vi "final Vi.vi"() -> ()   [LabVIEW 2018]
uses:
  <vilib>/Utility/file.llb/Read Delimited Spreadsheet (string).vi
  <vilib>/Utility/file.llb/Read Delimited Spreadsheet (DBL).vi
  <vilib>/Analysis/3filter.llb/Equi-Ripple BandPass (DBL).vi
  <vilib>/Analysis/NI_AALBase.lvlib
  <vilib>/Analysis/NI_AAL_SigProc.lvlib
panel:
  out "Locations 2":dbl[](array[numeric])
  out "yeee":dbl[](array[numeric])
  out "我們計算的RR":cluster{i32[], dbl[]}(graph)
  out "Array":dbl[](array[numeric])
  in  "threshold":dbl=10000.0 format="%0.2f"
  out "Locations":dbl[](array[numeric])
  in  "filter higher  stop freq":dbl(slide)=0.4094594594594595 scale=0.4..0.5
  out "平均心跳/分鐘":dbl
  out "?":bool
  out "RMSSD(ms)":dbl
  out "HR":cluster{i32[], dbl[]}[](graph)
  out "Mean R-R interval":dbl
  out "RR":cluster{dbl[], dbl[]}(graph)
  in  "filter lower stop freq":dbl(slide)=0.032972972972972976 scale=0.0..0.1
  out "Band filter":cluster{dbl[], "Filtered X":dbl[]}[](graph)
  out "Origin ECG":cluster{dbl[], i32[]}(graph)
  # "RMSSD越大，\n表示副交感神經作用越強"
  # "一般正常心跳約為50~100下/分鐘"
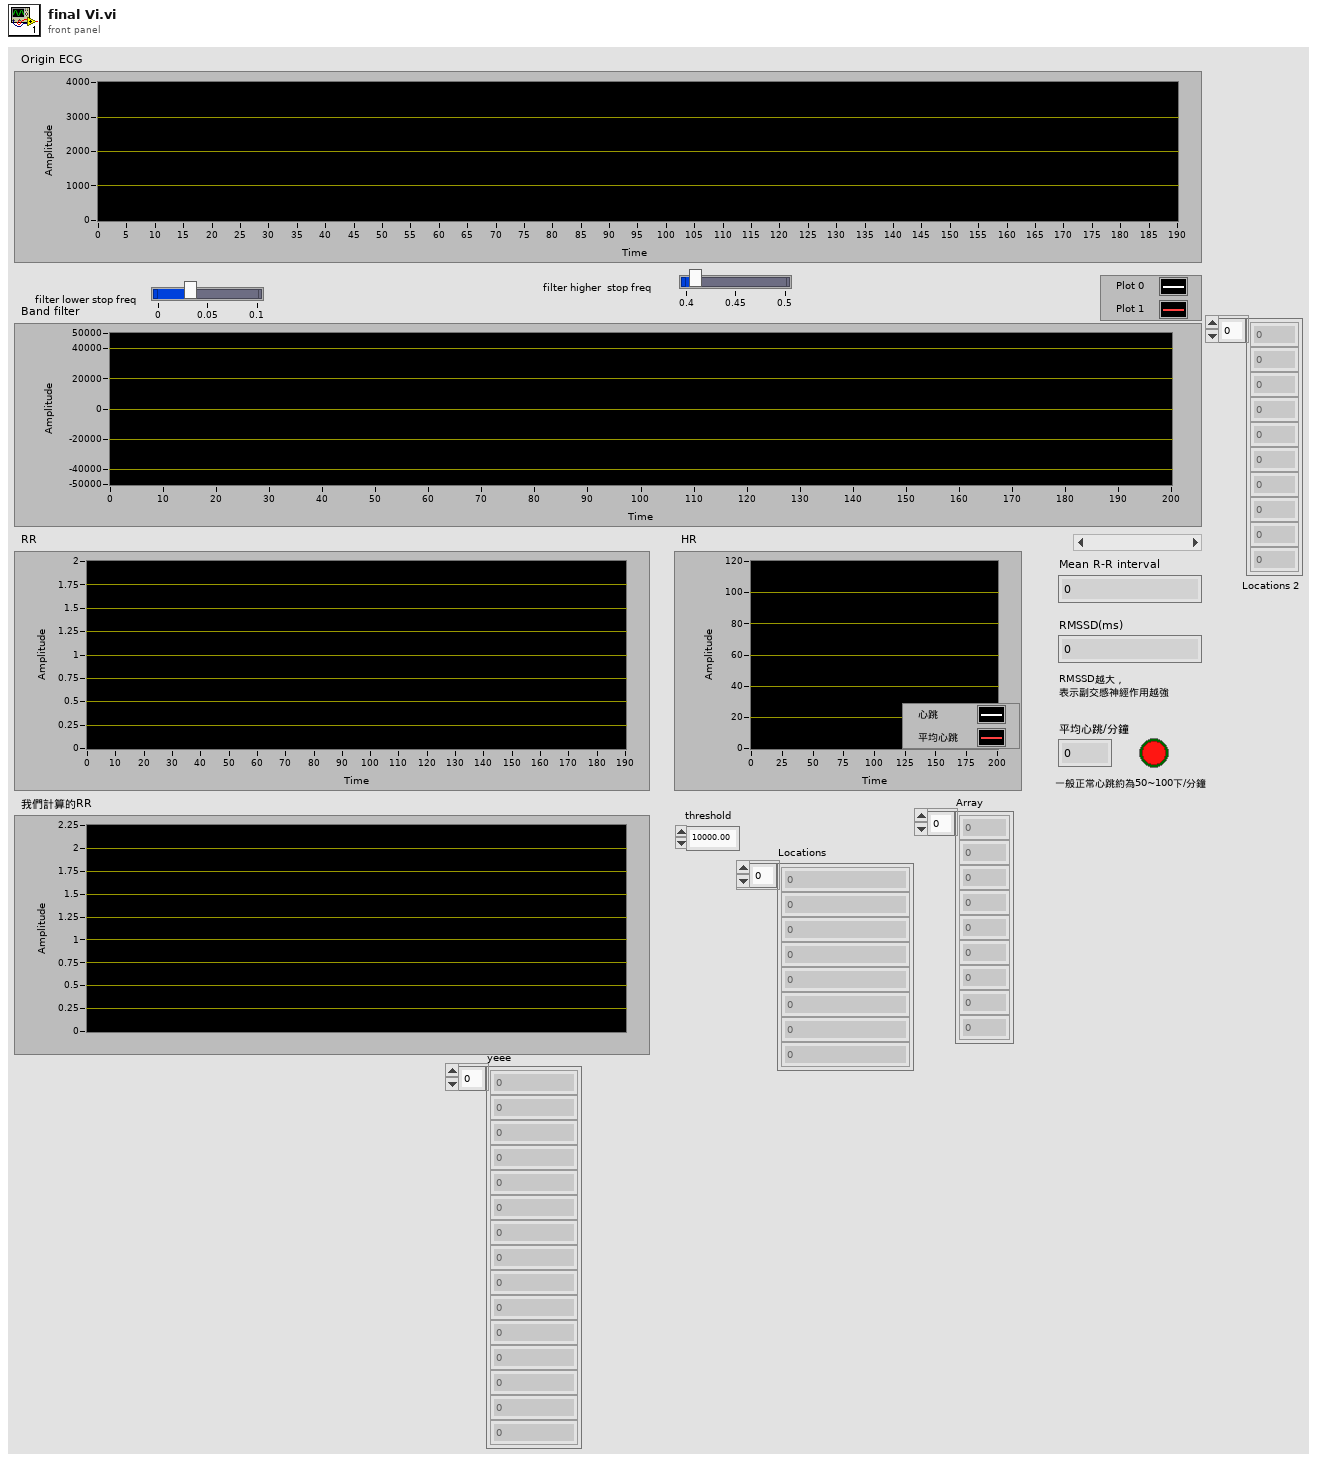
[diagram p1: front panel]
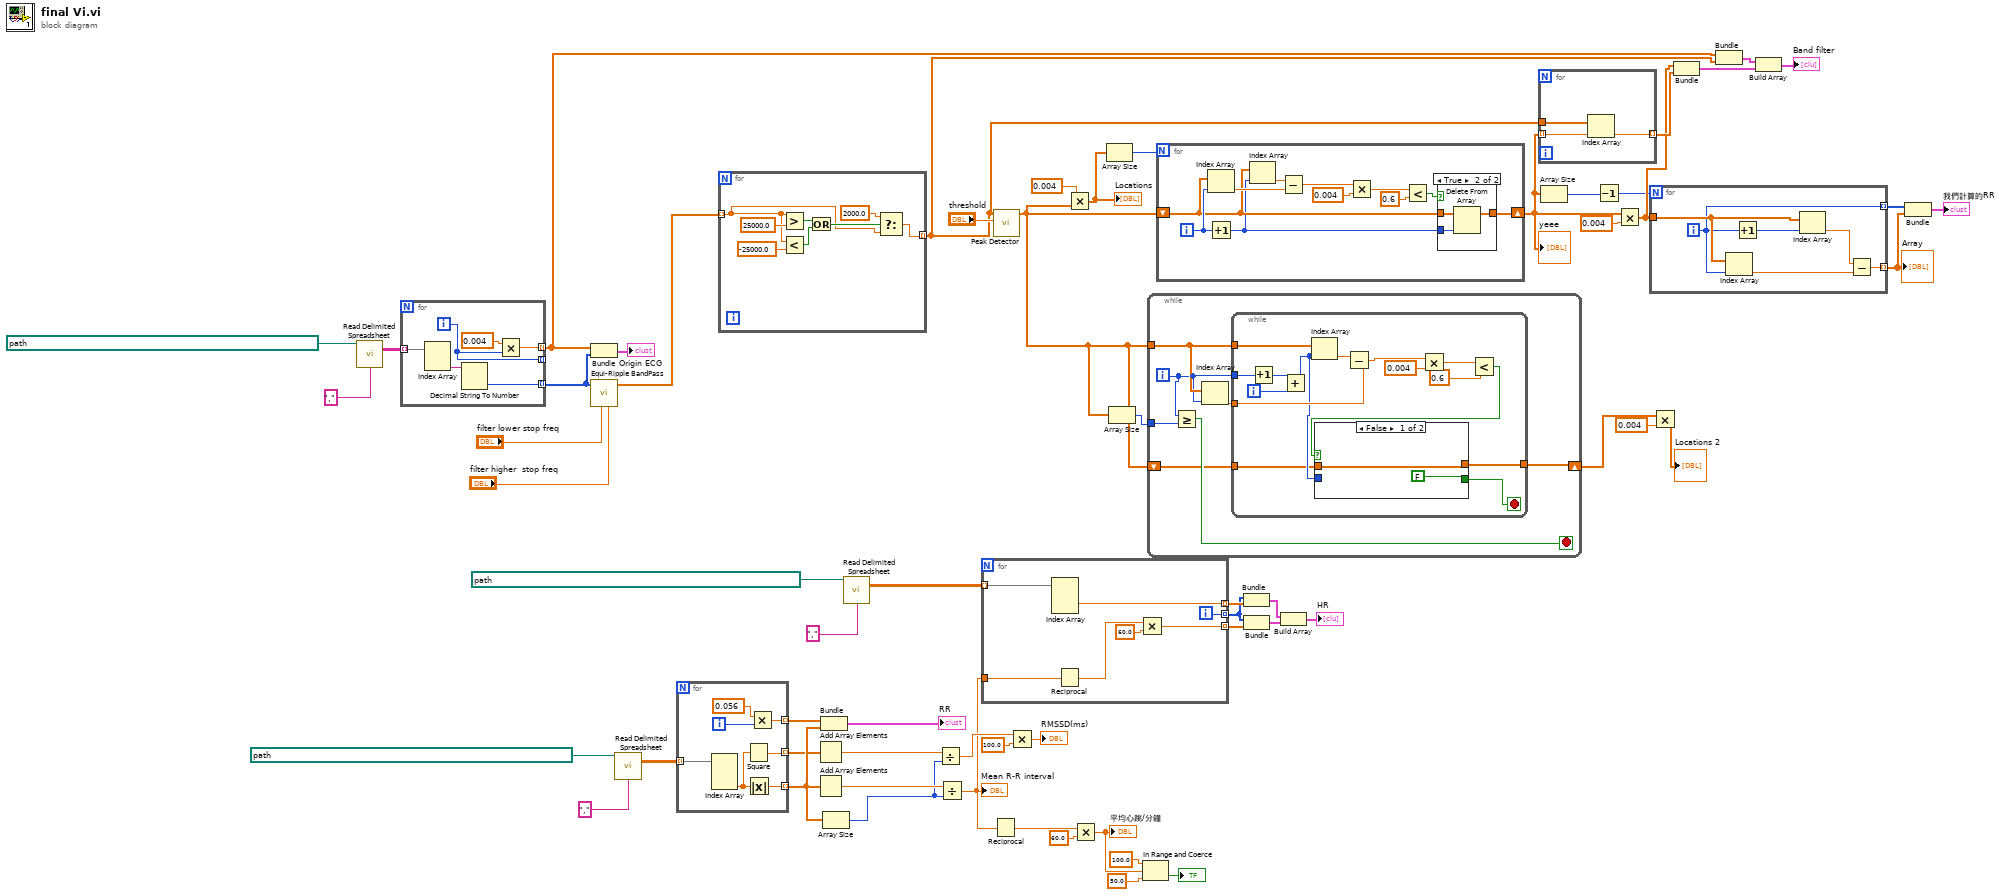
[diagram p0: block diagram]
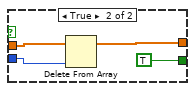
[diagram p2: hidden frame]
diagram:
  n1 = call-poly <vilib>:"Read Delimited Spreadsheet.vi"("file path (dialog if empty)"=path "D:/Documents/生醫儀表/data/2019_05_25__16_08_04_ECG.csv", "delimiter (\\t)"="," ("delimiter (\\t)")) -> ("all rows"=w59:string[][])  [unwired: 8 in, 5 out]
  n2 = for {
    tunnel: w59 -> [w66] mode=indexing
    tunnel: [w65] -> w23 mode=indexing
    tunnel: [w63] -> w17 mode=indexing
    tunnel: [w61] -> _ mode=indexing
    i -> [w61]
    n3 = Index Array(array=w66) -> (element #2=w62:string)  [unwired: 2 in, 1 out]
    n4 = Decimal String To Number(string=w62) -> (number=w65:i32)  [unwired: 2 in, 1 out]
    n5 = Multiply(x=0.004 ("y"), y=w61) -> (x*y=w63:dbl)
  }
  n6 = Bundle(w17, w23) -> (→"Origin ECG":cluster{dbl[], i32[]})  [unwired: 1 in]
  n7 = call-poly <vilib>:"Equi-Ripple BandPass.vi"("X"=w23, "lower stop freq"="filter lower stop freq", "higher stop freq"="filter higher  stop freq") -> ("Filtered X"=w9:dbl[])  [unwired: 5 in, 1 out]
  n8 = call-poly <vilib>:"Read Delimited Spreadsheet.vi"("file path (dialog if empty)"=path "D:/Documents/生醫儀表/data/2019_05_25__16_08_04_BR_RR.csv", "delimiter (\\t)"="," ("delimiter (\\t)")) -> ("all rows"=w56:dbl[][])  [unwired: 8 in, 5 out]
  n9 = for {
    tunnel: w56 -> [w73] mode=indexing
    tunnel: [w70] -> w54 mode=indexing
    tunnel: [w69] -> w50 mode=indexing
    tunnel: [w67] -> w40 mode=indexing
    i -> [w72]
    n10 = Index Array(array=w73) -> (element #3=w68:dbl)  [unwired: 3 in, 2 out]
    n11 = Square(x=w68) -> (x^2=w67:dbl)
    n12 = Absolute Value(x=w68) -> (abs(x)=w69:dbl)
    n13 = Multiply(x=0.056 ("y"), y=w72) -> (x*y=w70:dbl)
  }
  n14 = for {
    tunnel: w9 -> [w75] mode=indexing
    tunnel: [w74] -> w8 mode=indexing
    n15 = Greater?(x=w75, y=25000.0) -> (0:w79:bool)
    n16 = Less?(x=w75, y=-25000.0) -> (x < y?=w78:bool)
    n17 = Or(x=w79, y=w78) -> (x .or. y?=w77:bool)
    n18 = Select(t=2000.0, s=w77, f=w75) -> (s? t:f=w74:dbl)
  }
  n19 = Add Array Elements(numeric array=w40) -> (sum=w39:dbl)
  n20 = Add Array Elements(numeric array=w50) -> (sum=w51:dbl)
  n21 = Bundle(w54, w50) -> (→"RR":cluster{dbl[], dbl[]})  [unwired: 1 in]
  n22 = Array Size(array=w50) -> (size(s)=w38:i32)
  n23 = call-poly <vilib>:"Read Delimited Spreadsheet.vi"("file path (dialog if empty)"=path "D:/Documents/生醫儀表/data/2019_05_25__16_08_04_General.csv", "delimiter (\\t)"="," ("delimiter (\\t)")) -> ("all rows"=w47:dbl[][])  [unwired: 8 in, 5 out]
  n24 = Divide(x=w39, y=w38) -> (x/y=w37:dbl)
  n25 = Divide(x=w51, y=w38) -> (x/y=w32:dbl)
  "Mean R-R interval" <- w32
  n26 = for {
    tunnel: w47 -> [w88] mode=indexing
    tunnel: [w87] -> w46 mode=indexing
    tunnel: [w86] -> w45 mode=indexing
    tunnel: w32 -> [w85]
    tunnel: [w82] -> w41 mode=indexing
    i -> [w86]
    n27 = Index Array(array=w88) -> (element #2=w87:dbl)  [unwired: 3 in, 2 out]
    n28 = Reciprocal(x=w85) -> (1/x=w84:dbl)
    n29 = Multiply(x=w84, y=60.0) -> (x*y=w82:dbl)
  }
  n30 = Reciprocal(x=w32) -> (1/x=w34:dbl)
  n31 = call <vilib>:"Peak Detector.vi"("threshold"="threshold", "X"=w8) -> ("Locations"=w4:dbl[])  [unwired: 5 in, 4 out]
  n32 = Multiply(x=w37, y=100.0) -> (x*y=→"RMSSD(ms)":dbl)
  n33 = Multiply(x=0.004 ("y"), y=w4) -> (x*y=w14:dbl[])
  "Locations" <- w14
  n34 = Multiply(x=w34, y=60.0) -> (x*y=w31:dbl)
  "平均心跳/分鐘" <- w31
  n35 = Array Size(array=w14) -> (size(s)=w15:i32)
  n36 = Array Size(array=w4) -> (size(s)=w5:i32)
  n37 = In Range and Coerce(upper limit=100.0, x=w31, lower limit=50.0) -> (In Range?=→"?":bool)  [unwired: 1 out]
  n38 = while {
    tunnel: w4 -> [w94]
    tunnel: w5 -> [w92]
    shift-right: [w89] -> w2
    shift-left: w4 -> [w90]
    i -> [w93]
    stop <- w91 stop-if-true
    n39 = Greater Or Equal?(x=w93, y=w92) -> (x >= y?=w91:bool)
    n40 = Index Array(array=w94, index=w93) -> (element=w95:dbl)
    n41 = while {
      tunnel: w95 -> [w106]
      tunnel: w93 -> [w109]
      tunnel: w94 -> [w107]
      tunnel: w90 -> [w98]
      tunnel: [w97] -> w89
      i -> [w110]
      stop <- w96 stop-if-true
      n42 = Increment(x=w109) -> (x+1=w108:i32)
      n43 = Add(x=w108, y=w110) -> (x+y=w99:i32)
      n44 = Index Array(array=w107, index=w99) -> (element=w105:dbl)
      n45 = Subtract(x=w105, y=w106) -> (x-y=w101:dbl)
      n46 = Multiply(x=w101, y=0.004) -> (x*y=w104:dbl)
      n47 = Less?(x=w104, y=0.6) -> (x < y?=w100:bool)
      n48 = case shown="False" w100 {
        tunnel: w99 -> [_ w115]
        tunnel: w98 -> [w112 w116]
        tunnel: [w112 w114] -> w97
        tunnel: [FALSE TRUE] -> w96
        frame False {
        }
        frame True {
          n49 = Delete From Array(array=w116, index=w115) -> (array with subset deleted=w114:dbl[])  [unwired: 1 in, 1 out]
        }
      }
    }
  }
  n50 = for {
    N: w15 -> [_]
    shift-right: [w120] -> w6
    shift-left: w4 -> [w122]
    i -> [w127]
    n51 = Index Array(array=w122, index=w127) -> (element=w125:dbl)
    n52 = Increment(x=w127) -> (x+1=w121:i32)
    n53 = Index Array(array=w122, index=w121) -> (element=w126:dbl)
    n54 = Subtract(x=w126, y=w125) -> (x-y=w124:dbl)
    n55 = Multiply(x=w124, y=0.004) -> (x*y=w119:dbl)
    n56 = Less?(x=w119, y=0.6) -> (x < y?=w123:bool)
    n57 = case shown="True" w123 {
      tunnel: w122 -> [w128 w131]
      tunnel: w121 -> [_ w130]
      tunnel: [w128 w129] -> w120
      frame False {
      }
      frame True {
        n58 = Delete From Array(array=w131, index=w130) -> (array with subset deleted=w129:dbl[])  [unwired: 1 in, 1 out]
      }
    }
  }
  "yeee" <- w6
  n59 = Bundle(w45, w46) -> (w44:cluster{i32[], dbl[]})  [unwired: 1 in]
  n60 = Bundle(w45, w41) -> (w42:cluster{i32[], dbl[]})  [unwired: 1 in]
  n61 = Build Array(w44, w42) -> (→"HR":cluster{i32[], dbl[]}[])
  n62 = for {
    tunnel: w6 -> [w133] mode=indexing
    tunnel: w8 -> [w134]
    tunnel: [w132] -> w19 mode=indexing
    n63 = Index Array(array=w134, index=w133) -> (element=w132:dbl)
  }
  n64 = Array Size(array=w6) -> (size(s)=w11:i32)
  n65 = Decrement(x=w11) -> (x-1=w10:i32)
  n66 = Multiply(x=w6, y=0.004) -> (x*y=w12:dbl[])
  n67 = for {
    N: w10 -> [_]
    tunnel: w12 -> [w140]
    tunnel: [w136] -> w16 mode=indexing
    tunnel: [w135] -> w24 mode=indexing
    i -> [w135]
    n68 = Index Array(array=w140, index=w135) -> (element=w137:dbl)
    n69 = Increment(x=w135) -> (x+1=w139:i32)
    n70 = Index Array(array=w140, index=w139) -> (element=w138:dbl)
    n71 = Subtract(x=w138, y=w137) -> (x-y=w136:dbl)
  }
  "Array" <- w16
  n72 = Multiply(x=w2, y=0.004) -> (x*y=→"Locations 2":dbl[])
  n73 = Bundle(w12, w19) -> (w18:cluster{dbl[], dbl[]})  [unwired: 1 in]
  n74 = Bundle(w17, w8) -> (w21:cluster{dbl[], dbl[]})  [unwired: 1 in]
  n75 = Build Array(w21, w18) -> (→"Band filter":cluster{dbl[], dbl[]}[])
  n76 = Bundle(w24, w16) -> (→"我們計算的RR":cluster{i32[], dbl[]})  [unwired: 1 in]
